vi "critical.vi"(4 "defaultButton":T1 items=["NoButton"=0, "Ok"=1024, "Save"=2048, "SaveAll"=4096, "Open"=8192, "Yes"=16384, "YesToAll"=32768, "No"=65536, "NoToAll"=131072, "Abort"=262144, "Retry"=524288, "Ignore"=1048576, "Close"=2097152, "Cancel"=4194304, "Discard"=8388608, "Help"=16777216, "Apply"=33554432, "Reset"=67108864, "RestoreDefaults"=134217728], 5 "parent":refnum<class "QWidget.lvclass">, 6 "buttons":T1 items=["NoButton"=0, "Ok"=1024, "Save"=2048, "SaveAll"=4096, "Open"=8192, "Yes"=16384, "YesToAll"=32768, "No"=65536, "NoToAll"=131072, "Abort"=262144, "Retry"=524288, "Ignore"=1048576, "Close"=2097152, "Cancel"=4194304, "Discard"=8388608, "Help"=16777216, "Apply"=33554432, "Reset"=67108864, "RestoreDefaults"=134217728], 8 "Error In":errorcluster, 9 "text":string, 10 "title":string) -> (0 "Error Out":errorcluster, 2 "Value":T1 items=["NoButton"=0, "Ok"=1024, "Save"=2048, "SaveAll"=4096, "Open"=8192, "Yes"=16384, "YesToAll"=32768, "No"=65536, "NoToAll"=131072, "Abort"=262144, "Retry"=524288, "Ignore"=1048576, "Close"=2097152, "Cancel"=4194304, "Discard"=8388608, "Help"=16777216, "Apply"=33554432, "Reset"=67108864, "RestoreDefaults"=134217728])   [LabVIEW 2014, in "QMessageBox.lvclass"]
doc: "LabVIEW-specific documentation is not yet available. See <b>http://doc.qt.io/qt-5/QMessageBox.html#critical</b>"
uses:
  QMessageBox.lvclass
  StandardButton.ctl
  QWidget/QWidget.lvclass
  LQ Core/LQIdentity/LQIdentity.lvclass/LQIdentity.ctl
  LQ Core/LQ Core.lvlib
  LQ Core/LQIdentity/LQIdentity.lvclass
panel:
  # "Copyright (c) 2016 Sze Howe Koh\n\nThis Source Code Form is subject to the terms of the Mozilla Public\nLicense, v. 2.0. If a copy of the MPL was not distributed with this\nfile, You can obtain one at http://mozilla.org/MPL/2.0/."
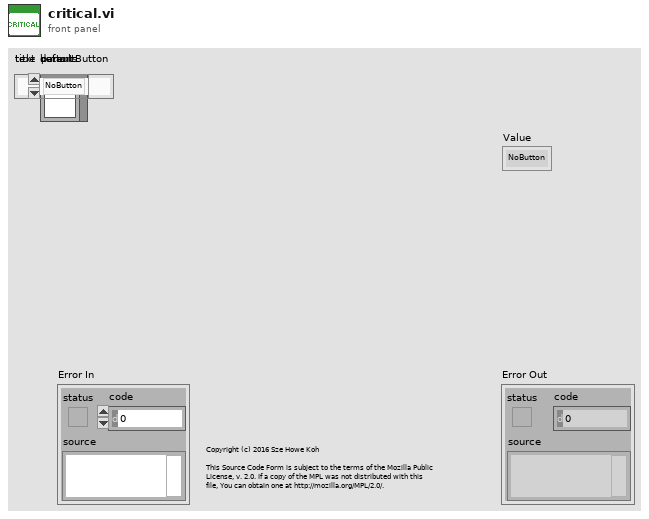
[diagram p1: front panel]
types:
  T1 = typedef "QMessageBox.lvclass/StandardButton.ctl" = i32
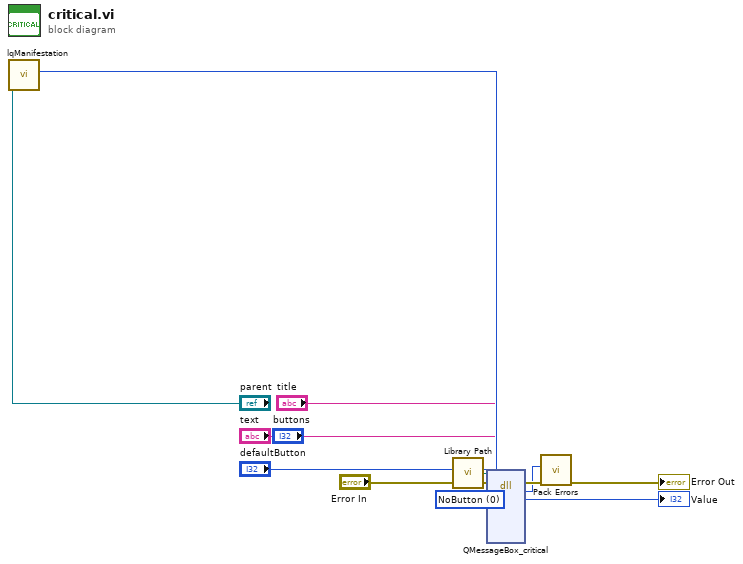
[diagram p0: block diagram]
diagram:
  w12 = T1 0 items=["NoButton"=0, "Ok"=1024, "Save"=2048, "SaveAll"=4096, "Open"=8192, "Yes"=16384, "YesToAll"=32768, "No"=65536, "NoToAll"=131072, "Abort"=262144, "Retry"=524288, "Ignore"=1048576, "Close"=2097152, "Cancel"=4194304, "Discard"=8388608, "Help"=16777216, "Apply"=33554432, "Reset"=67108864, "RestoreDefaults"=134217728] ("retVal")
  n1 = call "lqManifestation.vi"("LQIdentity in"="parent") -> ("Manifestation"=w5:u64)  [unwired: 9 in, 1 out]
  n2 = call "Library Path.vi"() -> ("Library Path"=w11:path)
  n3 = dll-call lib="?" fn="QMessageBox_critical"(path in=w11, error in="Error In", "_retVal"=w12, "parent"=w5, "title"="title", "text"="text", "buttons"="buttons", "defaultButton"="defaultButton") -> (error out=w9:errorcluster, w7:i32, "_retVal"=→"Value":i32)  [unwired: 6 in, 1 out]
  n4 = call "Pack Errors.vi"("Error In"=w9, "Error Code"=w7) -> ("Error Out"=→"Error Out":errorcluster)  [unwired: 9 in]
